vi "PH_Class.Generate Event.vi"(0 "i ref in":refnum<vi>, 2 "Class":string, 5 "error in (no error)":errorcluster) -> (14 "i ref out":refnum<vi>, 19 "error out":errorcluster)   [LabVIEW 2014, in "PH_Class.lvlib"]
uses:
  PH_Class.lvlib
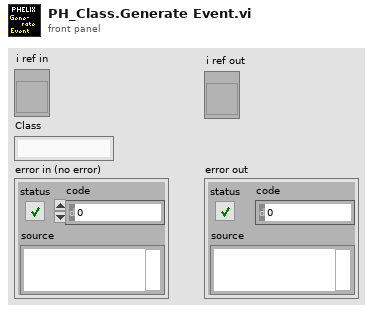
[diagram p1: front panel]
types:
  T1 = typedef "PH_Class.lvlib/PH_Class.i attribute.ctl" = cluster{"Event":refnum<user-event>, "Event registered":refnum<k4>, "GUI Refs stored":refnum<k4>}
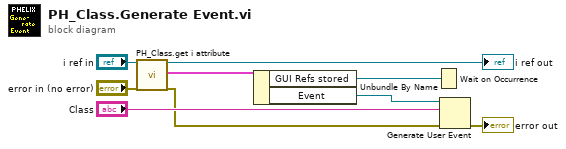
[diagram p0: block diagram]
diagram:
  n1 = call "PH_Class.get i attribute.vi"("i ref in"="i ref in", "error in (no error)"="error in (no error)") -> ("i ref out"=→"i ref out":refnum<vi>, "i attribute"=w6:T1, "error out"=w4:errorcluster)  [unwired: 15 in]
  n2 = Unbundle By Name(w6) -> ("GUI Refs stored"=w7:refnum<k4>, "Event"=w9:refnum<user-event>)
  n3 = Wait on Occurrence(2:w7) -> ()  [unwired: 2 in, 1 out]
  n4 = Generate User Event(user event=w9, event data cluster="Class", error in=w4) -> (error out=→"error out":errorcluster)  [unwired: 1 in, 1 out]
